vi "refgen_outer.vi"(11 "Qube":refnum<class "System.lvclass">) -> (3 "Qube":refnum<class "System.lvclass">)   [LabVIEW 2021, in "System.lvclass"]
uses:
  System.lvclass
  System.lvclass/System.ctl
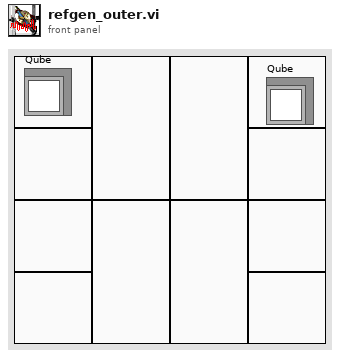
[diagram p1: front panel]
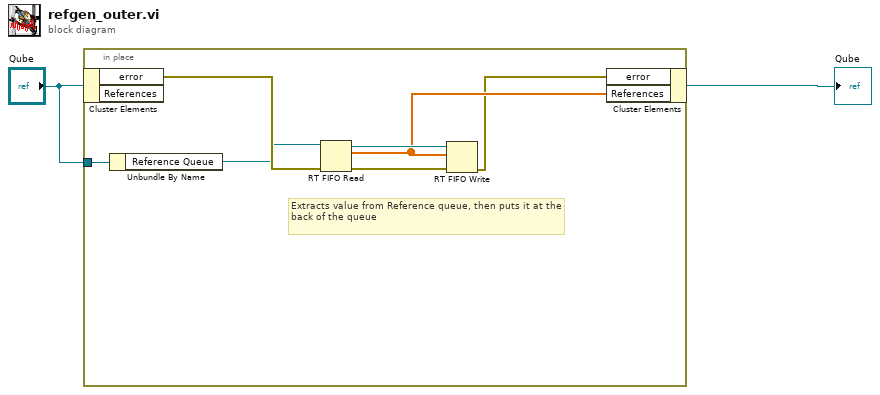
[diagram p0: block diagram]
diagram:
  n1 = in-place {
    in-place-border: "Qube" -> [w9]
    # "Extracts value from Reference queue, then puts it at the back of the queue"
    n2 = in-place-cluster #1("Qube") -> ("error"=w8:errorcluster)  [unwired: 1 out]
    n3 = Unbundle By Name(w9) -> ("Reference Queue"=w3:refnum<k33>)
    n4 = RT FIFO Read(0:w3, 3:w8) -> (8:w7:refnum<k33>, 9:w6:dbl[], 11:w5:errorcluster)  [unwired: 2 in, 2 out]
    n5 = RT FIFO Write(0:w7, 1:w6, 3:w5) -> (11:w4:errorcluster)  [unwired: 2 in, 3 out]
    n6 = in-place-cluster #1("error"=w4, "References"=w6) -> (→"Qube":refnum<class "System.lvclass">)
  }
